vi "GetAnalogCommand.vi"(1 "Pin":u8) -> (0 "Command":T1)   [LabVIEW 2021]
uses:
  CommandType.ctl
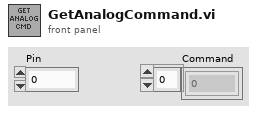
[diagram p1: front panel]
types:
  T1 = typedef "CommandType.ctl" = u8[]
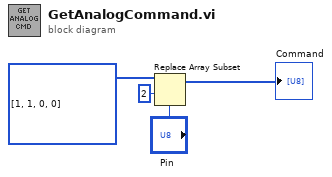
[diagram p0: block diagram]
diagram:
  n1 = Replace Array Subset(array=u8[] [1, 1, 0, 0], new element="Pin", index=2 ("indice")) -> (→"Command":u8[])
